vi "INIT SetECUProperties.vi"(7 "DB Alias data":T1, 8 "error in (no error)":errorcluster, 11 "Device Item Ref in":T2 format="%.0x") -> (0 "error out":errorcluster, 3 "Device Item Ref out":T2 format="%.0x")   [LabVIEW 2018, in "CAN Gateway System Explorer.lvlib"]
uses:
  CAN Gateway System Explorer.lvlib
  <vilib>/NI Veristand/Custom Device API/Custom Device Item Ref.ctl
  Types/Alias DB data.ctl
  Shared/Constants.vi
  <vilib>/NI Veristand/Custom Device API/Set Item Property (String).vi
  <vilib>/NI Veristand/Custom Device API/Custom Device API.lvlib
  Shared/CAN Gateway Shared.lvlib
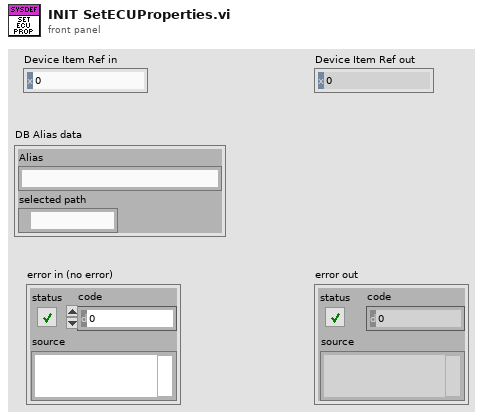
[diagram p1: front panel]
types:
  T1 = typedef "CAN Gateway System Explorer.lvlib/Alias DB data.ctl" = cluster{"Alias":string, "selected path":path}
  T2 = typedef "Custom Device API.lvlib/Custom Device Item Ref.ctl" = u64
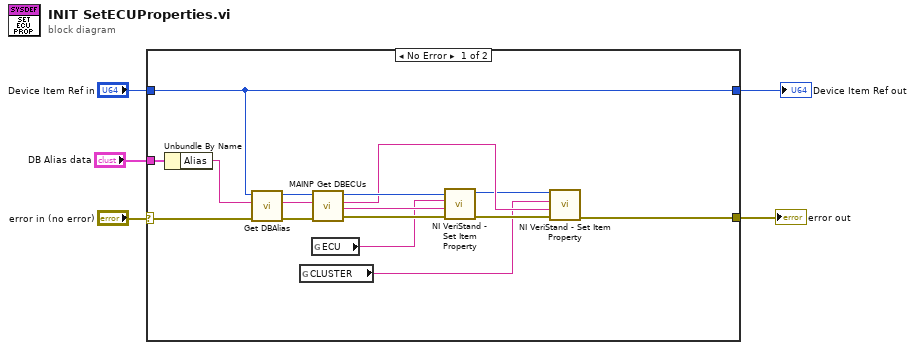
[diagram p0: block diagram]
diagram:
  n1 = case shown="No Error" "error in (no error)" {
    selector: "error in (no error)" -> [w20 w22]
    tunnel: "Device Item Ref in" -> [w19 w23]
    tunnel: [w21 w22] -> w3
    tunnel: [w19 w23] -> w2
    tunnel: "DB Alias data" -> [w8 _]
    frame No Error {
      n2 = Unbundle By Name(w8) -> ("Alias"=w7:string)
      n3 = call "Get DBAlias.vi"("error in (no error)"=w20, "DB Alias"=w7, "Device Item Ref in"=w19) -> ("error out"=w17:errorcluster, "Alias"=w6:string, "Device Item Ref out"=w18:T2)  [unwired: 6 in]
      n4 = global read "Constants.vi" "CLUSTER"() -> (w9:string)
      n5 = global read "Constants.vi" "ECU"() -> (w13:string)
      n6 = call "MAINP Get DBECUs.vi"("error in (no error)"=w17, "Alias"=w6, "Device Item Ref in"=w18) -> ("error out"=w15:errorcluster, "ECU"=w14:string, "Cluster"=w12:string, "Device Item Ref out"=w16:T2)  [unwired: 5 in]
      n7 = call-poly <vilib>:"NI VeriStand - Set Item Property.vi"("error in (no error)"=w15, "Value"=w14, "Property Name"=w13, "Item Ref in"=w16) -> ("error out"=w10:errorcluster, "Item Ref out"=w11:T2)  [unwired: 5 in, 1 out]
      n8 = call-poly <vilib>:"NI VeriStand - Set Item Property.vi"("error in (no error)"=w10, "Value"=w12, "Property Name"=w9, "Item Ref in"=w11) -> ("error out"=w21:errorcluster)  [unwired: 5 in, 2 out]
    }
    frame Error {
    }
  }
  "error out" <- w3
  "Device Item Ref out" <- w2
